vi "Script Msg Msg VI.vi"(4 "Name":string, 6 "Name Msg Refs.Msg VI":refnum<vi>, 8 "error in":errorcluster, 9 "Terminal Attributes (Init Msg Output)":T1, 10 "Terminal Attributes (Read Msg Input)":T1) -> (0 "error out":errorcluster)   [LabVIEW 2025, in "_Rescript.lvlib" / "Msg.lvlib" / "Msg.lvclass"]
uses:
  _Rescript/_Rescript.lvclass/_Rescript.ctl
  Msg.lvclass
  Msg.lvclass/Msg.ctl
  <vilib>/Utility/traverseref.llb/TRef TravTarget.ctl
  Attributes.ctl
  _Rescript.lvlib
  Terminal Attributes.ctl
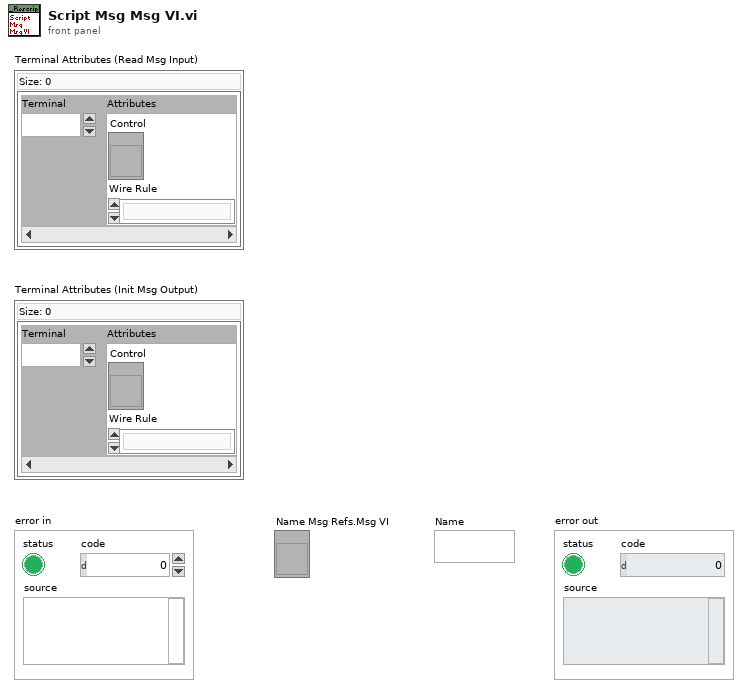
[diagram p1: front panel]
types:
  T1 = typedef "_Rescript.lvlib/Terminal Attributes.ctl" = map{i32, T2}
  T2 = typedef "_Rescript.lvlib/Attributes.ctl" = cluster{"Control":refnum<vi>, "Wire Rule":enum16{"Invalid Wire Rule", "Required", "Recommended", "Optional", "Dynamic Dispatch"}}
  T3 = typedef "TRef TravTarget.ctl" = enum16{"FP", "BD", "Other"}
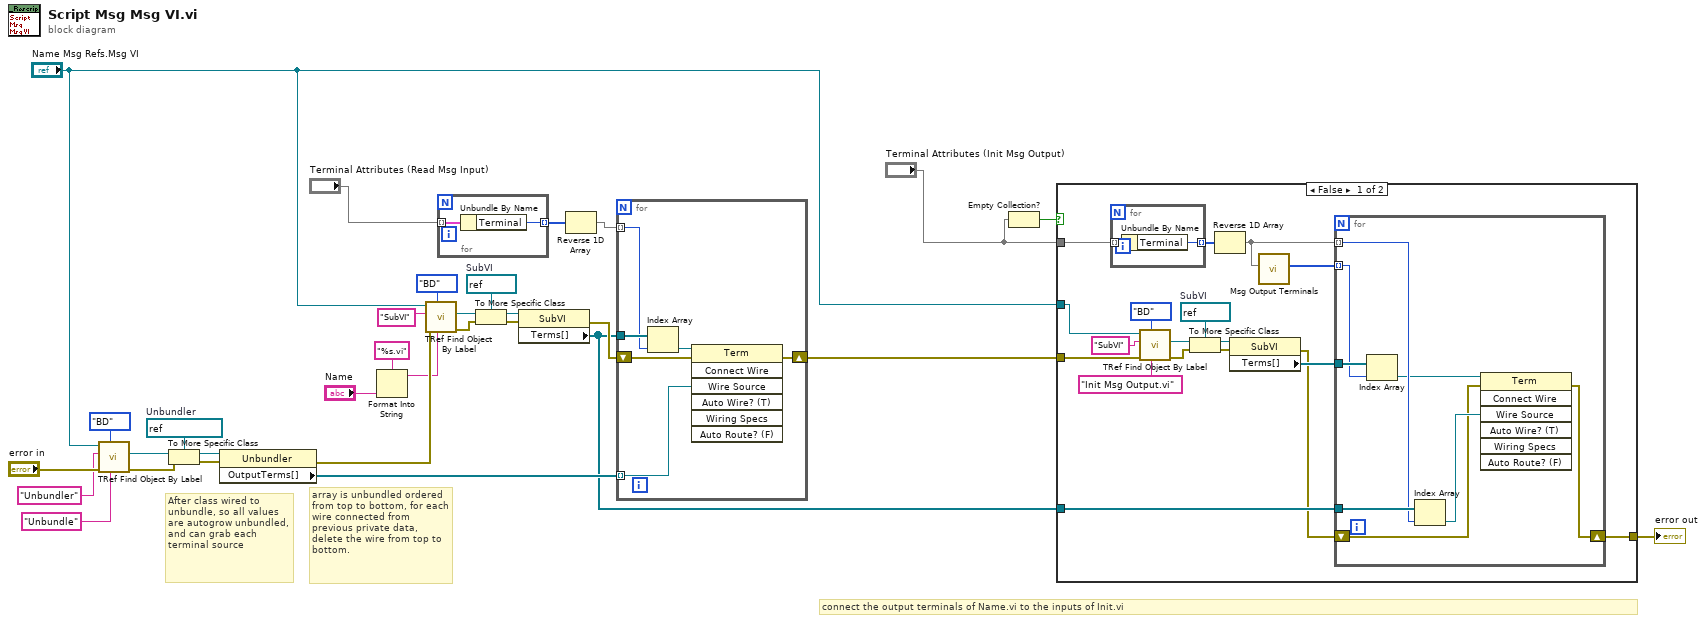
[diagram p0: block diagram]
diagram:
  w16 = refnum<vi> refnum  # Unbundler
  w30 = refnum<vi> refnum  # SubVI
  # "connect the output terminals of Name.vi to the inputs of Init.vi"
  # "array is unbundled ordered from top to bottom, for each wire connected from previous private data, delete the wire from top to bottom."
  # "After class wired to unbundle, so all values are autogrow unbundled, and can grab each terminal source"
  n1 = call <vilib>:"TRef Find Object By Label.vi"("Label"="Unbundle", "Traverse Target"=TRef_TravTarget."BD", "error in (no error)"="error in", "Class Name"="Unbundler", "VI Ref"="Name Msg Refs.Msg VI") -> ("error out"=w17:errorcluster, "Found Obj Ref"=w15:refnum<vi>)  [unwired: 3 in, 2 out]
  n2 = To More Specific Class(target class=w16, reference=w15, error in=w17) -> (specific class reference=w12:refnum<vi>, error out=w9:errorcluster)
  n3 = property class="Unbundler"(reference=w12, error in=w9) -> (error out=w21:errorcluster, "OutputTerms[]"=w8:refnum<vi>[])  [unwired: 1 out]
  n4 = Format Into String(format string="%s.vi", "Name") -> (resulting string=w18:string)  [unwired: 2 in, 1 out]
  n5 = call <vilib>:"TRef Find Object By Label.vi"("Label"=w18, "Traverse Target"=TRef_TravTarget."BD", "error in (no error)"=w21, "Class Name"="SubVI", "VI Ref"="Name Msg Refs.Msg VI") -> ("error out"=w29:errorcluster, "Found Obj Ref"=w20:refnum<vi>)  [unwired: 3 in, 2 out]
  n6 = for {
    tunnel: "Terminal Attributes (Read Msg Input)" -> [w33] mode=indexing
    tunnel: [w32] -> w25 mode=indexing
    n7 = Unbundle By Name(w33) -> ("Terminal"=w32:i32)
  }
  n8 = To More Specific Class(target class=w30, reference=w20, error in=w29) -> (specific class reference=w27:refnum<vi>, error out=w26:errorcluster)
  n9 = property class="SubVI"(reference=w27, error in=w26) -> (error out=w24:errorcluster, "Terms[]"=w6:refnum<vi>[])  [unwired: 1 out]
  n10 = Reverse 1D Array(array=w25) -> (reversed array=w22:i32[])
  n11 = for {
    tunnel: w6 -> [w39]
    tunnel: w22 -> [w38] mode=indexing
    shift-right: [w35] -> w3
    shift-left: w24 -> [w36]
    tunnel: w8 -> [w34] mode=indexing
    n12 = Index Array(array=w39, index=w38) -> (element=w37:refnum<vi>)
    n13 = invoke class="Term" method="Connect Wire"(reference=w37, error in=w36, "Wire Source"=w34) -> (error out=w35:errorcluster)  [unwired: 4 in, 6 out]
  }
  n14 = Empty Collection?(1:"Terminal Attributes (Init Msg Output)") -> (0:w7:bool)
  n15 = case shown="False" w7 {
    tunnel: "Terminal Attributes (Init Msg Output)" -> [w56 _]
    tunnel: w6 -> [w55 _]
    tunnel: [w54 w68] -> w5
    tunnel: "Name Msg Refs.Msg VI" -> [w46 _]
    tunnel: w3 -> [w44 w68]
    frame False {
      w52 = refnum<vi> refnum  # SubVI
      n16 = for {
        tunnel: w56 -> [w59] mode=indexing
        tunnel: [w58] -> w57 mode=indexing
        n17 = Unbundle By Name(w59) -> ("Terminal"=w58:i32)
      }
      n18 = call <vilib>:"TRef Find Object By Label.vi"("Label"="Init Msg Output.vi", "Traverse Target"=TRef_TravTarget."BD", "error in (no error)"=w44, "Class Name"="SubVI", "VI Ref"=w46) -> ("error out"=w51:errorcluster, "Found Obj Ref"=w48:refnum<vi>)  [unwired: 3 in, 2 out]
      n19 = To More Specific Class(target class=w52, reference=w48, error in=w51) -> (specific class reference=w50:refnum<vi>, error out=w49:errorcluster)
      n20 = Reverse 1D Array(array=w57) -> (reversed array=w41:i32[])
      n21 = property class="SubVI"(reference=w50, error in=w49) -> (error out=w43:errorcluster, "Terms[]"=w45:refnum<vi>[])  [unwired: 1 out]
      n22 = call "Msg Output Terminals.vi"("Msg Output Terminals"=w41) -> ("Init Msg Output Terminals"=w40:i32[])  [unwired: 9 in, 1 out]
      n23 = for {
        tunnel: w45 -> [w67]
        tunnel: w55 -> [w66]
        tunnel: w40 -> [w65] mode=indexing
        tunnel: w41 -> [w64] mode=indexing
        shift-right: [w60] -> w54
        shift-left: w43 -> [w61]
        n24 = Index Array(array=w67, index=w65) -> (element=w63:refnum<vi>)
        n25 = Index Array(array=w66, index=w64) -> (element=w62:refnum<vi>)
        n26 = invoke class="Term" method="Connect Wire"(reference=w63, error in=w61, "Wire Source"=w62) -> (error out=w60:errorcluster)  [unwired: 4 in, 6 out]
      }
    }
    frame True {
    }
  }
  "error out" <- w5
